vi "RelayPan.vi"(8 "error in (no error)":errorcluster caption="entrée d'erreur (pas d'erreur)", 11 "LSCI332.lvclass":refnum<class "LSCI332.lvclass">) -> (0 "error out":errorcluster caption="sortie d'erreur", 3 "LSCI332.lvclass Out":refnum<class "LSCI332.lvclass">)   [LabVIEW 2019, in "LSCI332.lvclass"]
uses:
  LSCI332.lvclass
  C:/Programmes Labview/LabscanV1A/DevicesClass/BaseDevice/BaseDevice.lvclass
  LSCI332.lvclass/LSCI332.ctl
  BaseDevice/ClassQueueMess.ctl
  BaseDevice/Accessor/GetClassEvent.vi
panel:
  out "R2 Func":string
  in  "Relay 2":bool
  out "R1 Func":string
  in  "Relay 1":bool
  in  "MainProgQEvent":refnum<user-event>
  in  "MainProgQ":refnum<queue>
  in  "Acq":bool
  in  "Stop":bool
  out "Init Program":bool
  # "Lakeshore 332"
  # "this MUST labeled with class name"
  # "this MUST be present and labeled \"Stop\""
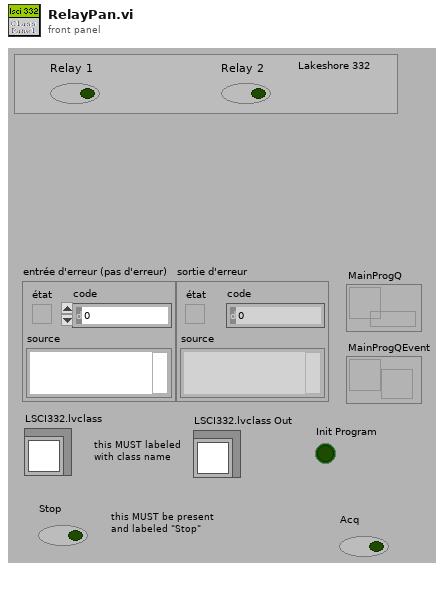
[diagram p1: front panel]
types:
  T1 = typedef "ClassQueueMess.ctl" = u16
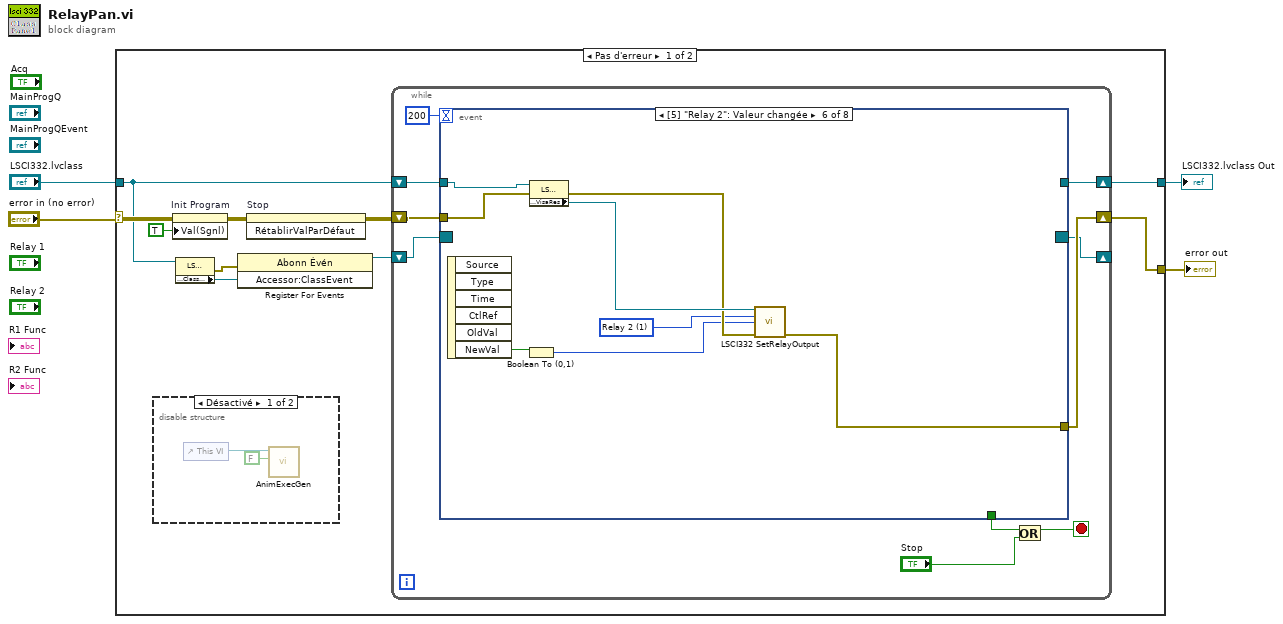
[diagram p0: block diagram]
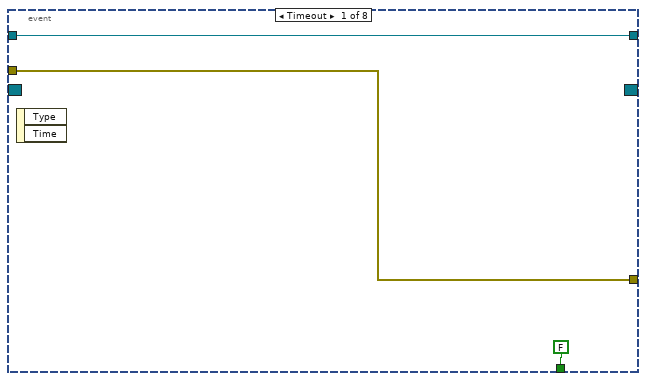
[diagram p3: hidden frame]
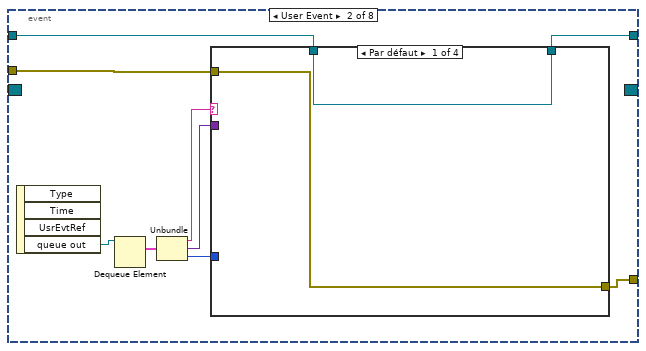
[diagram p4: hidden frame]
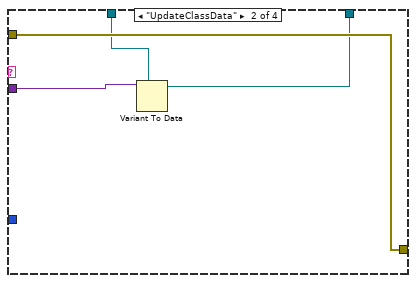
[diagram p5: hidden frame]
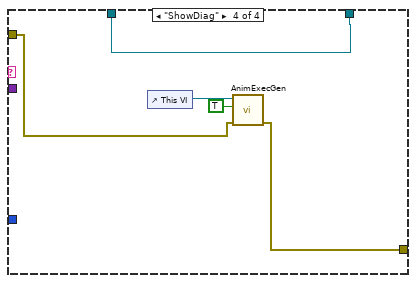
[diagram p7: hidden frame]
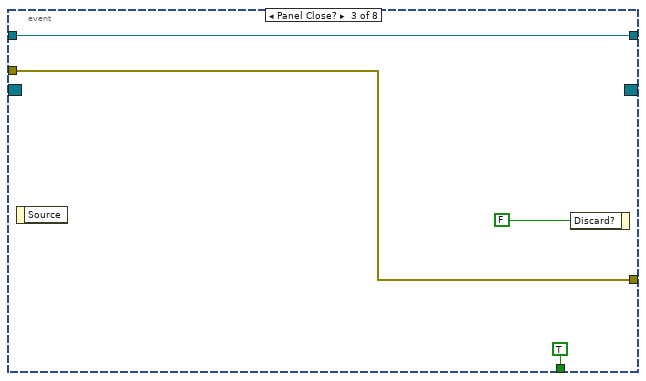
[diagram p8: hidden frame]
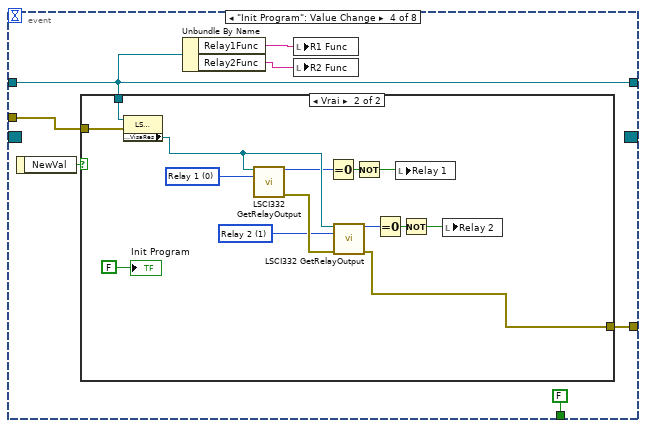
[diagram p9: hidden frame]
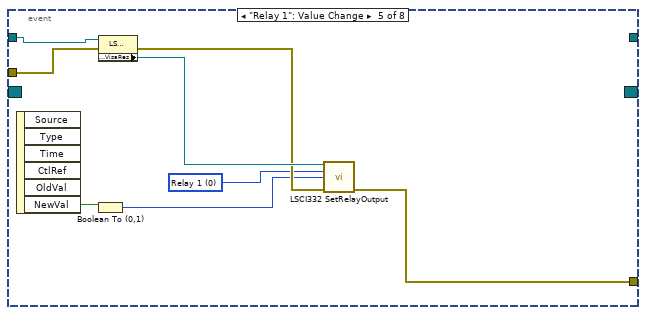
[diagram p11: hidden frame]
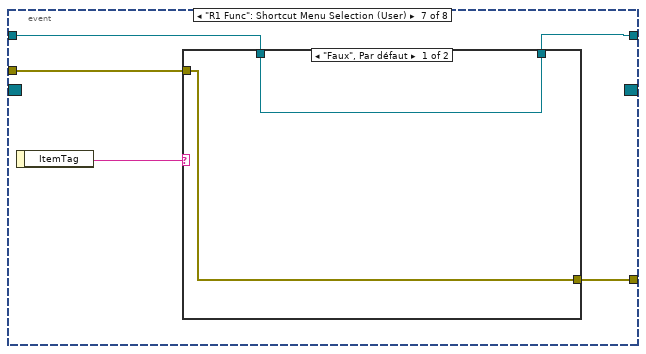
[diagram p12: hidden frame]
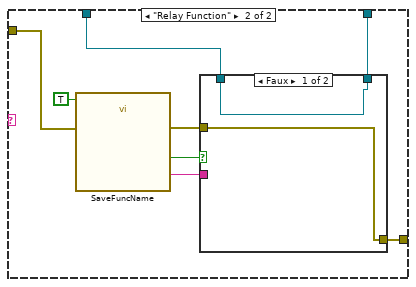
[diagram p13: hidden frame]
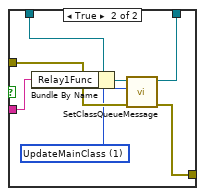
[diagram p14: hidden frame]
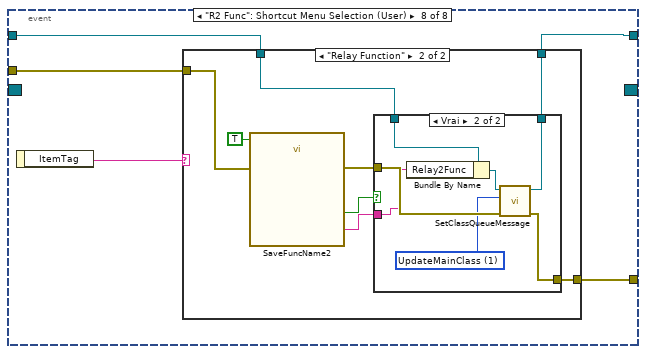
[diagram p15: hidden frame]
diagram:
  n1 = case shown="Pas d'erreur" "error in (no error)" {
    selector: "error in (no error)" -> [w11 w143]
    tunnel: [w14 w143] -> w3
    tunnel: "LSCI332.lvclass" -> [w6 w142]
    tunnel: [w12 w142] -> w1
    frame No Error {
      n2 = disable-structure shown="Désactivé" {
        frame Disabled {
          n3 = control-ref of="This VI"() -> (w15:refnum<vi>)
          n4 = call <userlib>:"AnimExecGen.vi"("Animer l'exécution ?"=FALSE, "ViRef"=w15) -> ()  [unwired: 9 in, 1 out]
        }
        frame Enabled {
        }
      }
      n5 = property on="Init Program" class="Bool (strict)"(error in=w11, "Val(Sgnl)"=TRUE ("Valeur (Signalisation)")) -> (error out=w10:errorcluster)  [unwired: 1 in, 1 out]
      n6 = property class="LSCI332.lvclass"(reference=w6) -> (error out=w8:errorcluster, "Accessor:ClassEvent"=w7:refnum<user-event>)  [unwired: 1 in, 1 out]
      n7 = register-events(error in=w8, w7) -> (reference out=w5:refnum<event-registration>)  [unwired: 1 in, 1 out]
      n8 = invoke on="Stop" class="Bool (strict)" method="RétablirValParDéfaut"(error in=w10) -> (error out=w9:errorcluster)  [unwired: 2 in, 2 out]
      n9 = while {
        shift-right: [w24] -> w14
        shift-left: w9 -> [w25]
        shift-right: [w21] -> w12
        shift-left: w6 -> [w23]
        shift-right: [w17] -> _
        shift-left: w5 -> [w18]
        stop <- w20 stop-if-true
        n10 = event shown="[5] \"Relay 2\": Valeur changée" {
          selector: w18 -> [_ _ _ _ _ _ _ _]
          dyn-events: [_ _ _ _ _ _ _ _] -> w17
          timeout: 200 -> [_ _ _ _ _ _ _ _]
          tunnel: w25 -> [w27 w37 w53 w61 w82 w90 w97 w121]
          tunnel: [w27 w31 w53 w60 w81 w89 w95 w119] -> w24
          tunnel: w23 -> [w28 w38 w52 w58 w85 w93 w96 w120]
          tunnel: [FALSE _ TRUE FALSE _ _ _ _] -> w22
          tunnel: [w28 w30 w52 w58 _ _ w94 w118] -> w21
          event Timeout {
            n11 = event-data() -> ()  [unwired: 1 in, 2 out]
          }
          event User Event {
            n12 = event-data() -> ("queue out"=w35:refnum<queue>)  [unwired: 1 in, 3 out]
            n13 = Dequeue Element(queue=w35) -> (element=w36:cluster{"Message":string, "Data":variant, i32})  [unwired: 2 in, 3 out]
            n14 = Unbundle(w36) -> ("Message"=w34:string, "Data"=w33:variant, w32:i32)
            n15 = case shown="Par défaut" w34 {
              tunnel: w37 -> [w40 w44 w45 w49]
              tunnel: w33 -> [_ w43 _ _]
              tunnel: w38 -> [w39 w42 w46 w47]
              tunnel: [w39 w41 w46 w47] -> w30
              tunnel: [w40 w44 w45 w48] -> w31
              tunnel: w32 -> [_ _ _ _]
              frame Default {
              }
              frame "UpdateClassData" {
                n16 = Variant To Data(type=w42, Variant=w43) -> (data=w41:refnum<class "LSCI332.lvclass">)  [unwired: 1 in, 1 out]
              }
              frame "MeasDone" {
              }
              frame "ShowDiag" {
                n17 = control-ref of="This VI"() -> (w50:refnum<vi>)
                n18 = call <userlib>:"AnimExecGen.vi"("ErrorIn(No Error)"=w49, "Animer l'exécution ?"=TRUE, "ViRef"=w50) -> ("sortie d'erreur"=w48:errorcluster)  [unwired: 8 in]
              }
            }
          }
          event Panel Close? {
            n19 = event-data() -> ()  [unwired: 1 in, 1 out]
            n20 = event-data("Discard?"=FALSE ("Rejeter ?")) -> ()  [unwired: 1 in, 1 out]
          }
          event "Init Program": Value Change {
            n21 = event-data() -> ("NewVal"=w62:bool)  [unwired: 1 in]
            n22 = case shown="Vrai" w62 {
              tunnel: w61 -> [w63 w75]
              tunnel: [w63 w64] -> w60
              tunnel: w58 -> [_ w76]
              frame False {
              }
              frame True {
                w72 = u32 1 items=["Relay 1", "Relay 2"] ("Relay(1)")
                w74 = u32 0 items=["Relay 1", "Relay 2"] ("Relay(1)")
                n23 = property class="LSCI332.lvclass"(reference=w76, error in=w75) -> ("Accessor:VisaRes"=w71:refnum<visa-resource-name>)  [unwired: 2 out]
                n24 = call <userlib>:"LSCI332 GetRelayOutput.vi"("VISA Rsrc"=w71, "Relay(1)"=w74) -> ("RelayMode"=w70:enum16{"Off", "On", "Alarm"}, "error out"=w73:errorcluster)  [unwired: 10 in, 2 out]
                n25 = Equal To 0?(x=w70) -> (x = 0?=w69:bool)
                n26 = call <userlib>:"LSCI332 GetRelayOutput.vi"("VISA Rsrc"=w71, "Relay(1)"=w72, "error in"=w73) -> ("RelayMode"=w65:enum16{"Off", "On", "Alarm"}, "error out"=w64:errorcluster)  [unwired: 9 in, 2 out]
                n27 = Not(x=w69) -> (.not. x?=w68:bool)
                n28 = Equal To 0?(x=w65) -> (x = 0?=w66:bool)
                n29 = local write "Relay 1"(w68) -> ()
                n30 = Not(x=w66) -> (.not. x?=w67:bool)
                n31 = local write "Relay 2"(w67) -> ()
                "Init Program" <- FALSE
              }
            }
            n32 = Unbundle By Name(w58) -> ("Relay1Func"=w56:string, "Relay2Func"=w57:string)
            n33 = local write "R1 Func"(w56) -> ()
            n34 = local write "R2 Func"(w57) -> ()
          }
          event "Relay 1": Value Change {
            w80 = u32 0 items=["Relay 1", "Relay 2"] ("Relay(1)")
            n35 = event-data() -> ("NewVal"=w79:bool)  [unwired: 1 in, 5 out]
            n36 = Boolean To (0,1)(Boolean=w79) -> (0, 1=w78:i16)
            n37 = property class="LSCI332.lvclass"(reference=w85, error in=w82) -> (error out=w83:errorcluster, "Accessor:VisaRes"=w84:refnum<visa-resource-name>)  [unwired: 1 out]
            n38 = call <userlib>:"LSCI332 SetRelayOutput.vi"("VISA Rsrc"=w84, "Relay(1)"=w80, "RelayMode"=w78, "error in"=w83) -> ("error out"=w81:errorcluster)  [unwired: 11 in]
          }
          event "Relay 2": Value Change {
            w88 = u32 1 items=["Relay 1", "Relay 2"] ("Relay(1)")
            n39 = event-data() -> ("NewVal"=w87:bool)  [unwired: 1 in, 5 out]
            n40 = Boolean To (0,1)(Boolean=w87) -> (0, 1=w86:i16)
            n41 = property class="LSCI332.lvclass"(reference=w93, error in=w90) -> (error out=w91:errorcluster, "Accessor:VisaRes"=w92:refnum<visa-resource-name>)  [unwired: 1 out]
            n42 = call <userlib>:"LSCI332 SetRelayOutput.vi"("VISA Rsrc"=w92, "Relay(1)"=w88, "RelayMode"=w86, "error in"=w91) -> ("error out"=w89:errorcluster)  [unwired: 11 in]
          }
          event "R1 Func": Shortcut Menu Selection (User) {
            n43 = event-data() -> ("ItemTag"=w98:string)  [unwired: 1 in]
            n44 = case shown="\"Faux\", Par défaut" w98 {
              tunnel: w97 -> [w99 w107]
              tunnel: w96 -> [w100 w101]
              tunnel: [w99 w103] -> w95
              tunnel: [w100 w102] -> w94
              frame "Faux", Default {
              }
              frame "Relay Function" {
                n45 = call "SaveFuncName"("Enable"=TRUE, "error in (no error)"=w107) -> ("Name"=w104:string, "Save"=w106:bool, "error out"=w105:errorcluster)  [unwired: 15 in]
                n46 = case shown="Faux" w106 {
                  tunnel: w101 -> [w109 w114]
                  tunnel: w105 -> [w110 w117]
                  tunnel: w104 -> [_ w112]
                  tunnel: [w110 w116] -> w103
                  tunnel: [w109 w115] -> w102
                  frame False {
                  }
                  frame True {
                    w111 = T1 1 items=["UpdateClassData", "UpdateMainClass"] ("Menu déroulant")
                    n47 = Bundle By Name(cluster=w114, "Relay1Func"=w112) -> (w113:refnum<class "LSCI332.lvclass">)
                    n48 = call-dynamic "SetClassQueueMessage.vi"("ErrorIn(No Error)"=w117, "Menu déroulant"=w111, "DefaultDev.lvclass"=w113) -> ("sortie d'erreur"=w116:errorcluster, "DefaultDev.lvclass Out"=w115:refnum<class "LSCI332.lvclass">)  [unwired: 7 in]
                  }
                }
              }
            }
          }
          event "R2 Func": Shortcut Menu Selection (User) {
            n49 = event-data() -> ("ItemTag"=w122:string)  [unwired: 1 in]
            n50 = case shown="\"Relay Function\"" w122 {
              tunnel: w121 -> [w123 w131]
              tunnel: w120 -> [w124 w125]
              tunnel: [w123 w127] -> w119
              tunnel: [w124 w126] -> w118
              frame "Faux", Default {
              }
              frame "Relay Function" {
                n51 = call "SaveFuncName2"("Enable"=TRUE, "error in (no error)"=w131) -> ("Name"=w128:string, "Save"=w130:bool, "error out"=w129:errorcluster)  [unwired: 15 in]
                n52 = case shown="Vrai" w130 {
                  tunnel: w125 -> [w133 w137]
                  tunnel: w129 -> [w134 w141]
                  tunnel: w128 -> [_ w138]
                  tunnel: [w134 w140] -> w127
                  tunnel: [w133 w139] -> w126
                  frame False {
                  }
                  frame True {
                    w135 = T1 1 items=["UpdateClassData", "UpdateMainClass"] ("Menu déroulant")
                    n53 = Bundle By Name(cluster=w137, "Relay2Func"=w138) -> (w136:refnum<class "LSCI332.lvclass">)
                    n54 = call-dynamic "SetClassQueueMessage.vi"("ErrorIn(No Error)"=w141, "Menu déroulant"=w135, "DefaultDev.lvclass"=w136) -> ("sortie d'erreur"=w140:errorcluster, "DefaultDev.lvclass Out"=w139:refnum<class "LSCI332.lvclass">)  [unwired: 7 in]
                  }
                }
              }
            }
          }
        }
        n55 = Or(x=w22, y="Stop") -> (x .or. y?=w20:bool)
      }
    }
    frame Error {
    }
  }
  "error out" <- w3
  "LSCI332.lvclass Out" <- w1
